vi "isDisabled.vi"(8 "error in (no error)":errorcluster, 11 "Transaction in":refnum<class "Transaction.lvclass">) -> (0 "error out":errorcluster, 2 "Disabled?":bool, 3 "Transaction out":refnum<class "Transaction.lvclass">)   [LabVIEW 2020, in "Transaction.lvclass"]
uses:
  Transaction.lvclass
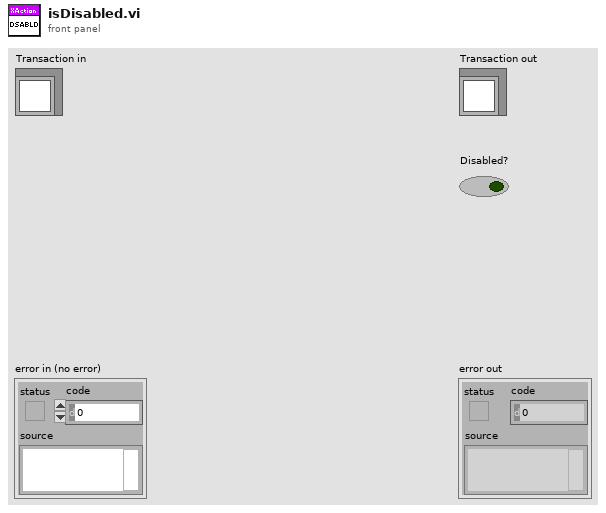
[diagram p1: front panel]
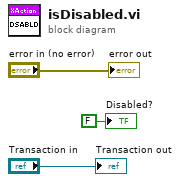
[diagram p0: block diagram]
diagram:
  "error out" <- "error in (no error)"
  "Transaction out" <- "Transaction in"
  "Disabled?" <- FALSE ("Disabled?")
